vi "path_input.vi"() -> (0 "Path input":path caption="selected path")   [LabVIEW 2016]
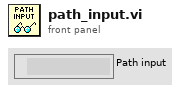
[diagram p1: front panel]
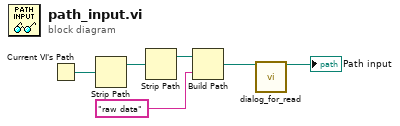
[diagram p0: block diagram]
diagram:
  n1 = Current VI's Path() -> (path=w1:path)
  n2 = Strip Path(path=w1) -> (stripped path=w2:path)  [unwired: 1 out]
  n3 = Strip Path(path=w2) -> (stripped path=w6:path)  [unwired: 1 out]
  n4 = Build Path(base path=w6, name or relative path="raw data") -> (appended path=w4:path)
  n5 = call "dialog_for_read.vi"("start path"=w4) -> ("selected path"=→"Path input":path)  [unwired: 11 in, 3 out]
